vi "Controller Main Loop.vi"(8 "error in (no error)":errorcluster, 11 "msg cluster":T1) -> (0 "error out":errorcluster)   [LabVIEW 2020]
uses:
  Messaging/Messaging Cluster.ctl
  Hardware/Sensors/Cameras/Camera.lvclass
  C:/Users/Haslach/Documents/Inflation-Apparatus/src/Hardware/General Hardware.lvclass
  Hardware/Sensors/Force Sensors/Force Sensor.lvclass
  Hardware/Actuators/Servos/Servo.lvclass
  Hardware/Actuators/Switches/Switch.lvclass
  Controller Loop/Message and Data.ctl
  Inflation Test/Parameter Class/IA Test Parameters.lvclass
  Controllers/Controller.lvclass
  File Interfacing/Filename Structure.ctl
  GUI/Main GUI Loop/Handler.ctl
  Inflation Test/Result Handling/Inflation Test Numeric Results.ctl
  Controller Loop/Controller Data.ctl
  Hardware/General Hardware.lvclass/General Hardware.ctl
  Hardware/General Hardware.lvclass
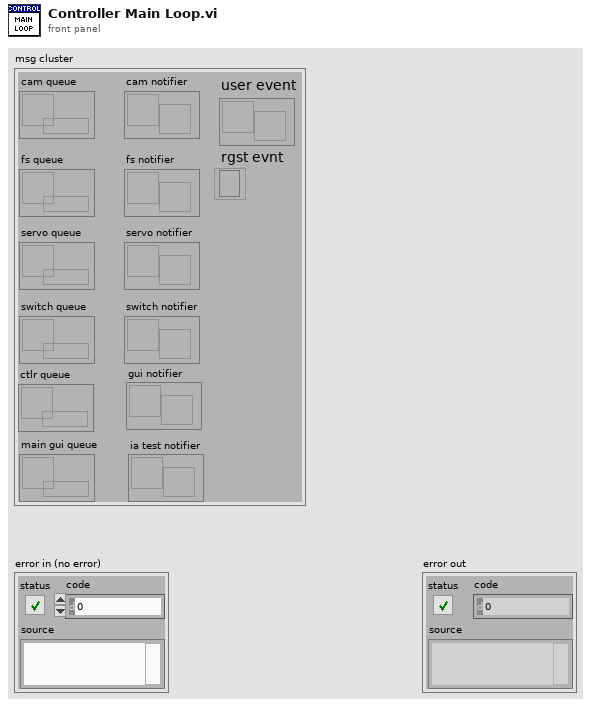
[diagram p1: front panel]
types:
  T1 = typedef "Messaging Cluster.ctl" = cluster{"cam queue":refnum<queue>, "fs queue":refnum<queue>, "servo queue":refnum<queue>, "switch queue":refnum<queue>, "switch notifier":refnum<notifier>, "servo notifier":refnum<notifier>, "fs notifier":refnum<notifier>, "cam notifier":refnum<notifier>, "rgst evnt":refnum<event-registration>, "user event":refnum<user-event>, "ctlr queue":refnum<queue>, "main gui queue":refnum<queue>, "gui notifier":refnum<notifier>, "ia test notifier":refnum<notifier>}
  T2 = typedef "Controller Data.ctl" = cluster{"diameter results":dbl[][], "force results":dbl[][], "fs cal array":dbl[][], "fs cal results":dbl[][], "start time":timestamp, "end time":timestamp, "log row":i32, "log column":i32}
  T3 = typedef "Handler.ctl" = cluster{"bool ref":refnum<vi>, "error":errorcluster, "msg":string, "status":string, "switch status":bool, "force cal":dbl[][], "force cal results":dbl[][]}
  T4 = enum32{"invalid app kind", "Development System", "Run Time System", "Student Edition", "Embedded LabVIEW", "Evaluation", "Custom"}
  T5 = typedef "Message and Data.ctl" = cluster{"msg":string, "ia test param":refnum<class "IA Test Parameters.lvclass">, "controller type":refnum<class "Controller.lvclass">, "folder path":path, "file name":string, "file comments":string, "cam":refnum<class "Camera.lvclass">, "fs":refnum<class "Force Sensor.lvclass">, "servo":refnum<class "Servo.lvclass">, "switch":refnum<class "Switch.lvclass">, "filename struct":T6}
  T6 = typedef "Filename Structure.ctl" = enum16{"<nameYYYYMMDDi>", "<name>"}
  T7 = typedef "Inflation Test Numeric Results.ctl" = cluster{"diameter":dbl, "diam time":dbl, "force":dbl, "force time":dbl, "setpoint":dbl, "servo pw":dbl, "calibration log":dbl[][], "calibration results":dbl[][]}
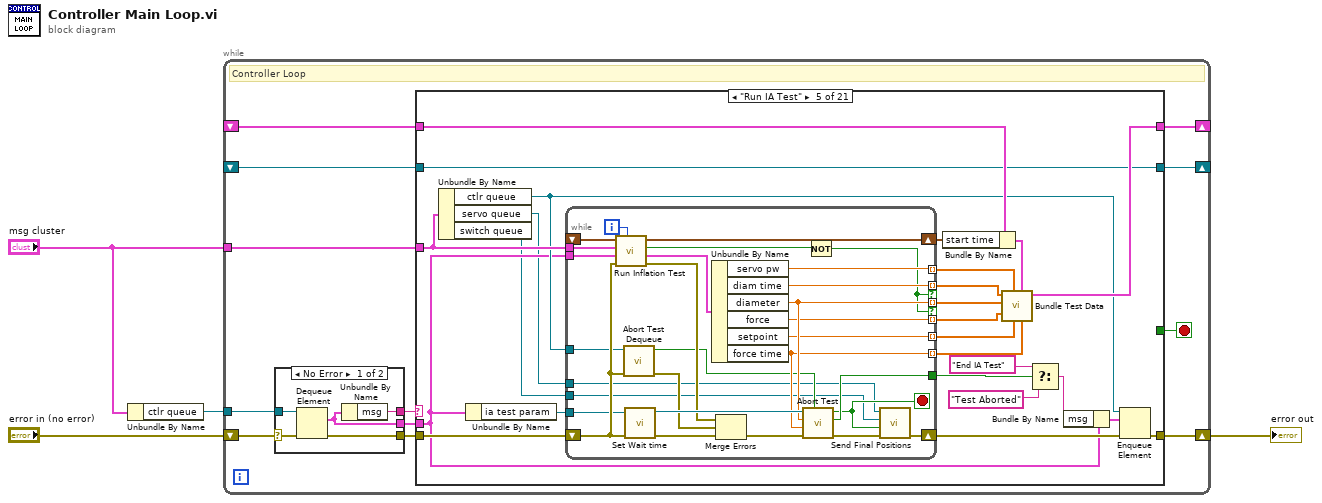
[diagram p0: block diagram]
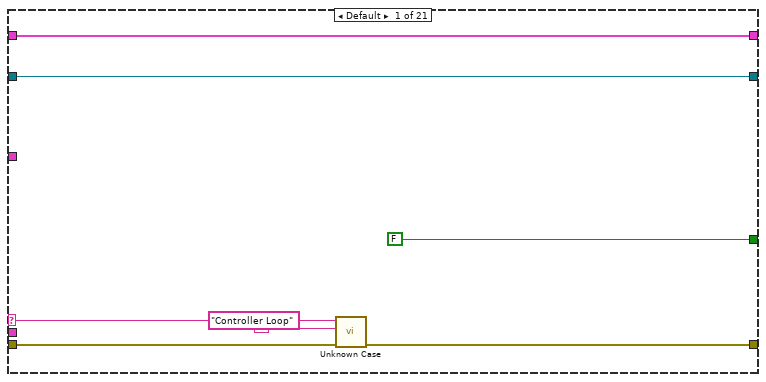
[diagram p2: hidden frame]
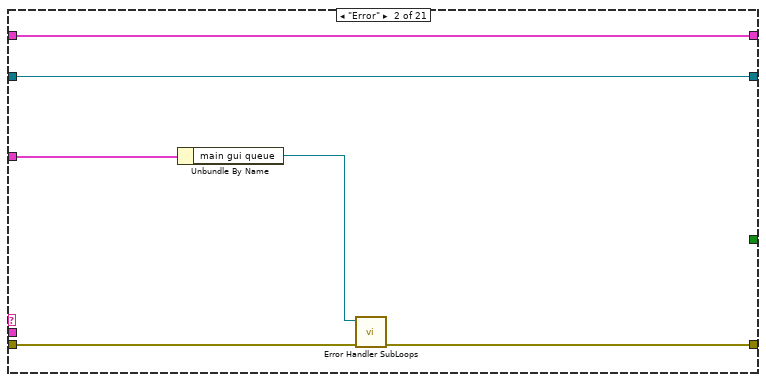
[diagram p3: hidden frame]
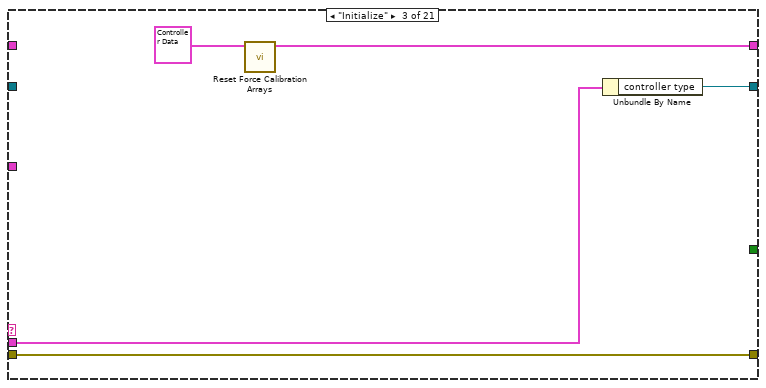
[diagram p4: hidden frame]
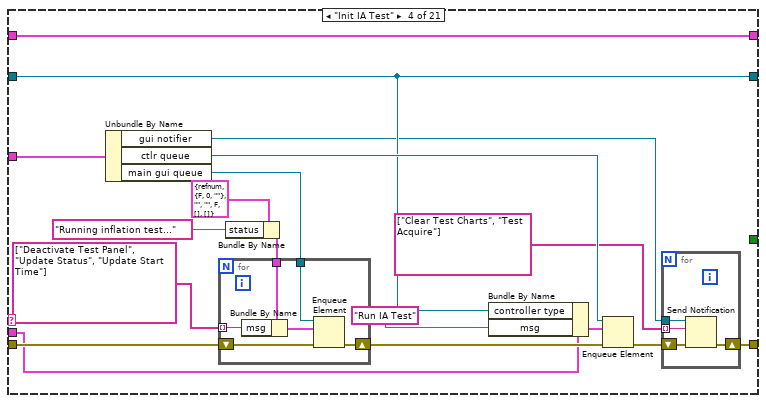
[diagram p5: hidden frame]
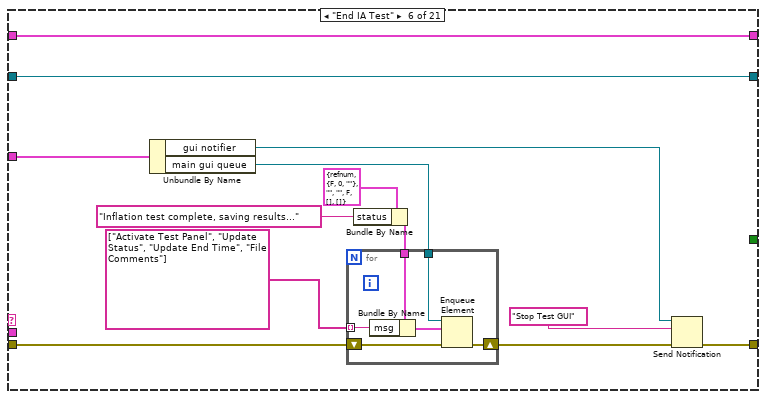
[diagram p6: hidden frame]
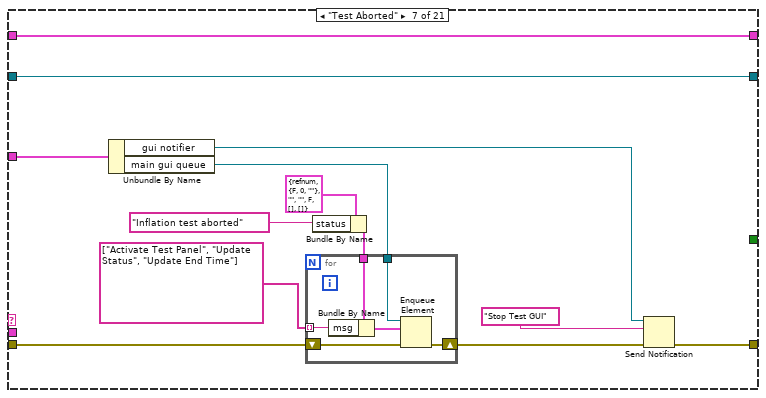
[diagram p7: hidden frame]
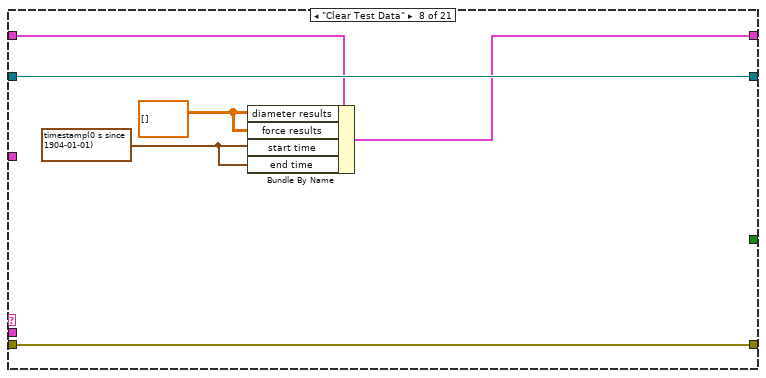
[diagram p8: hidden frame]
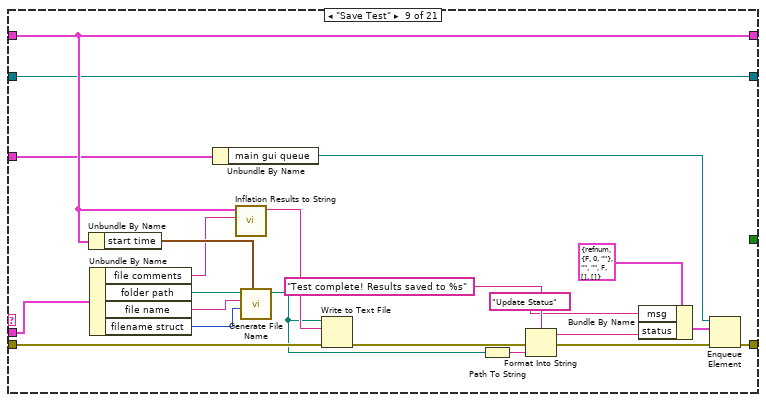
[diagram p9: hidden frame]
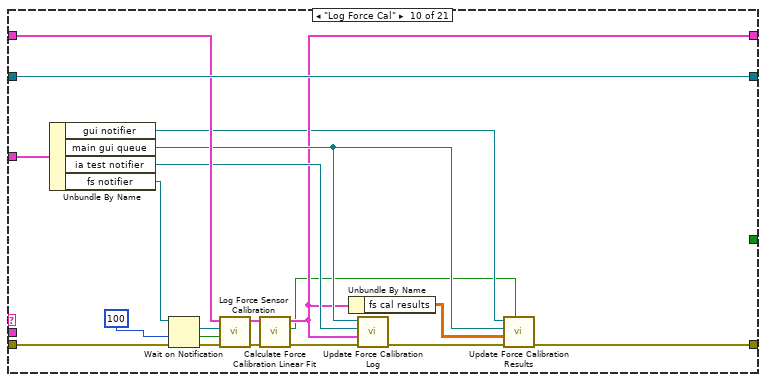
[diagram p10: hidden frame]
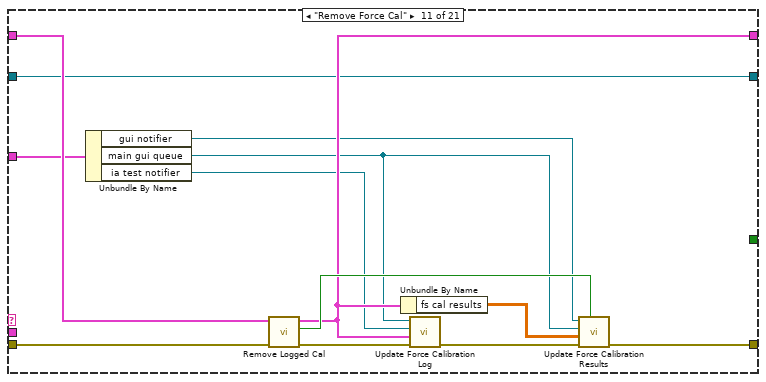
[diagram p11: hidden frame]
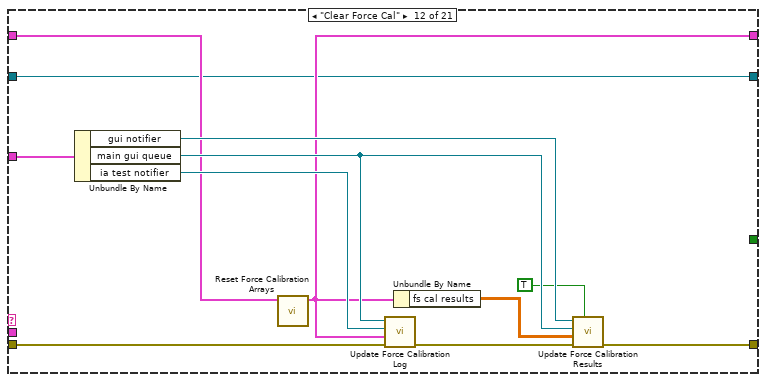
[diagram p12: hidden frame]
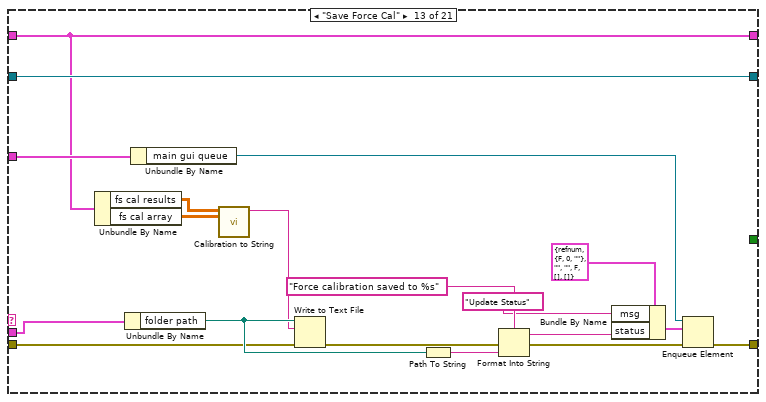
[diagram p13: hidden frame]
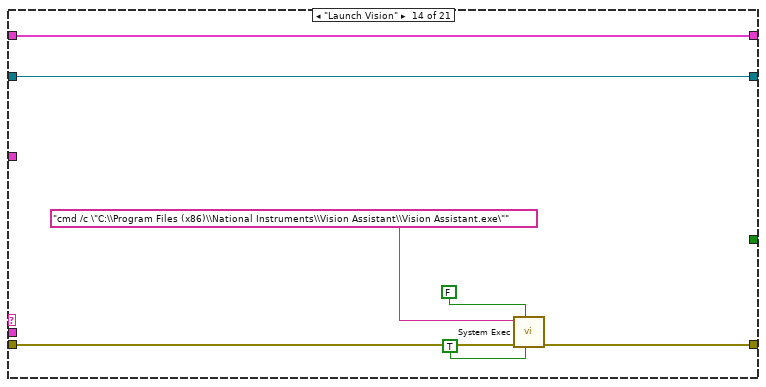
[diagram p14: hidden frame]
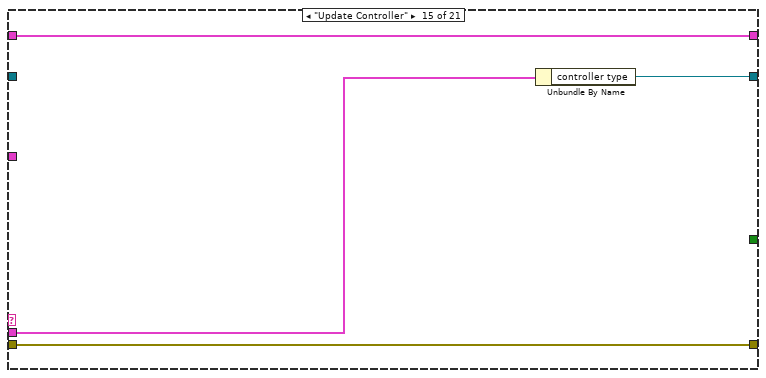
[diagram p15: hidden frame]
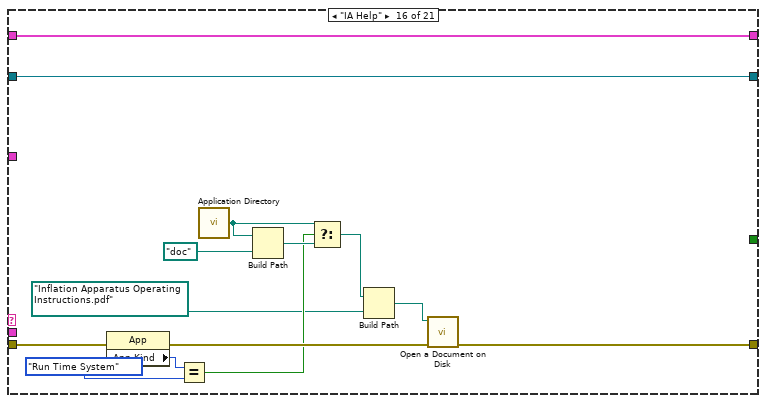
[diagram p16: hidden frame]
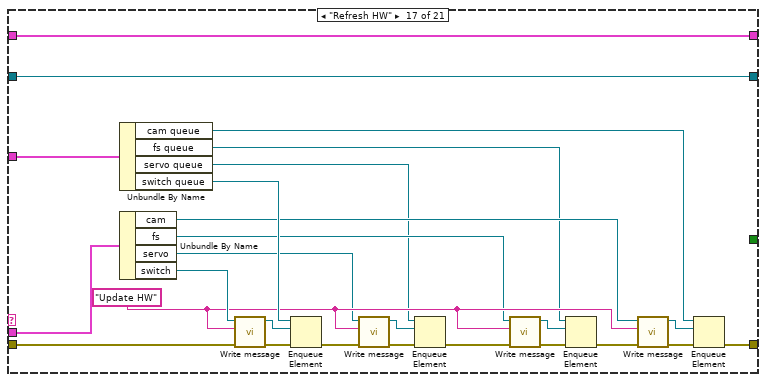
[diagram p17: hidden frame]
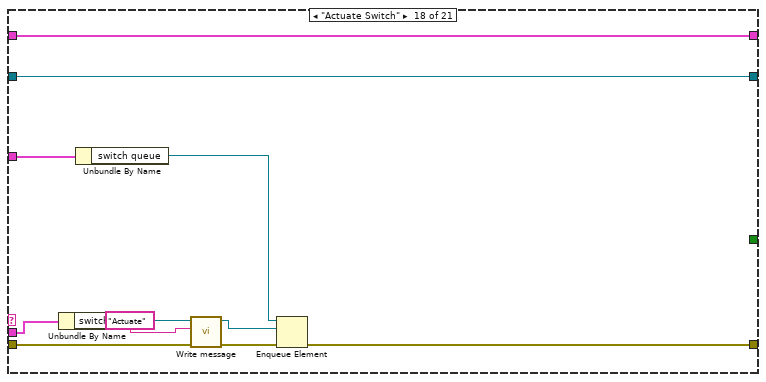
[diagram p18: hidden frame]
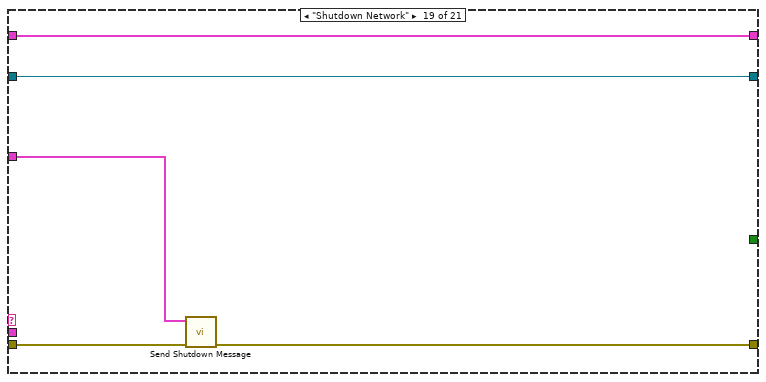
[diagram p19: hidden frame]
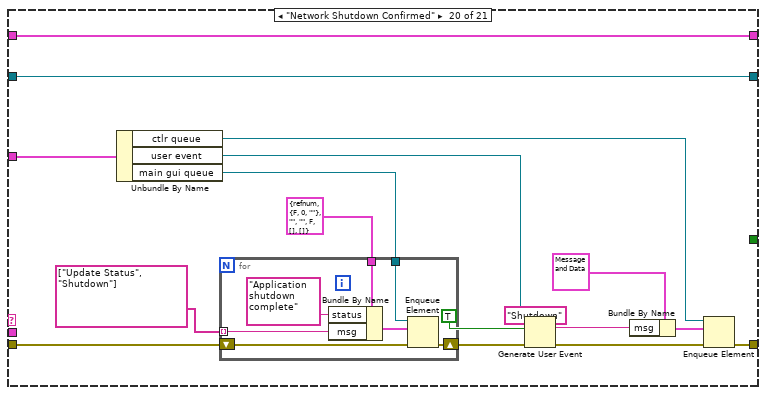
[diagram p20: hidden frame]
diagram:
  n1 = Unbundle By Name("msg cluster") -> ("ctlr queue"=w1:refnum<queue>)
  n2 = while {
    tunnel: "msg cluster" -> [w12]
    shift-right: [w14] -> w3
    shift-left: "error in (no error)" -> [w16]
    shift-right: [w8] -> _
    shift-left: _ -> [w9]
    tunnel: w1 -> [w7]
    shift-right: [w6] -> _
    shift-left: _ -> [w5]
    stop <- w11 stop-if-true
    # "Controller Loop"
    n3 = case shown="No Error" w16 {
      selector: w16 -> [w344 w348]
      tunnel: [w345 w348] -> w15
      tunnel: w7 -> [w343 _]
      tunnel: [w342 "Error" ("msg")] -> w13
      tunnel: [w341 T5 {"msg"="", "ia test param"=refnum, "controller type"=refnum, "folder path"=path "", "file name"="", "file comments"="", "cam"=refnum, "fs"=refnum, "servo"=refnum, "switch"=refnum, "filename struct"=enum."<nameYYYYMMDDi>"} ("controller loop")] -> w10
      frame No Error {
        n4 = Dequeue Element(queue=w343, error in (no error)=w344) -> (element=w341:T5, error out=w345:errorcluster)  [unwired: 1 in, 2 out]
        n5 = Unbundle By Name(w341) -> ("msg"=w342:string)
      }
      frame Error {
      }
    }
    n6 = case shown="\"Run IA Test\"" w13 {
      selector: w13 -> [w21 _ _ _ _ _ _ _ _ _ _ _ _ _ _ _ _ _ _ _ _]
      tunnel: w15 -> [w23 w26 w34 w50 w87 w125 w144 w155 w177 w199 w213 w226 w236 w250 w254 w266 w292 w303 w311 w327 w339]
      tunnel: [w22 w27 w34 w38 w72 w119 w138 w155 w167 w184 w207 w225 w230 w249 w254 w269 w279 w304 w312 w329 w339] -> w14
      tunnel: w12 -> [_ w29 _ w51 w76 w124 w143 _ w169 w202 w206 w224 w235 _ _ _ w294 w306 w313 w328 _]
      tunnel: [FALSE _ _ _ _ _ _ _ _ _ _ _ _ _ _ _ _ _ _ _ TRUE] -> w11
      tunnel: w10 -> [_ _ w33 w43 w70 _ _ _ w181 _ _ _ w238 _ w257 _ w297 w301 _ _ _]
      tunnel: w9 -> [w18 w28 _ w52 w79 w122 w141 w159 w178 w195 w211 w220 w228 w253 w255 w271 w295 w308 w310 w324 w338]
      tunnel: [w18 w28 w30 w52 w81 w122 w141 w156 w178 w187 w209 w217 w228 w253 w255 w271 w295 w308 w310 w324 w338] -> w8
      tunnel: [w17 w24 w32 w40 w75 w123 w142 w160 w175 w196 w208 w216 w229 w252 w256 w270 w296 w307 w309 w317 w337] -> w6
      tunnel: w5 -> [w17 w24 _ w40 w75 w123 w142 w160 w175 w196 w208 w216 w229 w252 _ w270 w296 w307 w309 w317 w337]
      frame Default {
        n7 = call "Unknown Case.vi"("error in (no error)"=w23, "source"="Controller Loop", "case"=w21) -> ("error out"=w22:errorcluster)  [unwired: 8 in]
      }
      frame "Error" {
        n8 = Unbundle By Name(w29) -> ("main gui queue"=w25:refnum<queue>)
        n9 = call "Error Handler SubLoops.vi"("error in"=w26, "main gui queue"=w25) -> ("error out"=w27:errorcluster)  [unwired: 9 in]
      }
      frame "Initialize" {
        n10 = call "Reset Force Calibration Arrays.vi"("array results in"=T2 {"diameter results"=[], "force results"=[], "fs cal array"=[], "fs cal results"=[], "start time"=timestamp(0 s since 1904-01-01), "end time"=timestamp(0 s since 1904-01-01), "log row"=0, "log column"=0} ("array results")) -> ("array results out"=w30:T2)  [unwired: 10 in]
        n11 = Unbundle By Name(w33) -> ("controller type"=w32:refnum<class "Controller.lvclass">)
      }
      frame "Init IA Test" {
        n12 = Unbundle By Name(w51) -> ("gui notifier"=w37:refnum<notifier>, "ctlr queue"=w44:refnum<queue>, "main gui queue"=w49:refnum<queue>)
        n13 = Bundle By Name(cluster=T3 {"bool ref"=refnum, "error"={"status"=FALSE, "code"=0, "source"=""}, "msg"="", "status"="", "switch status"=FALSE, "force cal"=[], "force cal results"=[]} ("main gui type"), "status"="Running inflation test...") -> (w46:T3)
        n14 = for {
          tunnel: w46 -> [w61]
          tunnel: w49 -> [w58]
          shift-right: [w60] -> w45
          shift-left: w50 -> [w62]
          tunnel: string[] ["Deactivate Test Panel", "Update Status", "Update Start Time"] ("msg") -> [w57] mode=indexing
          n15 = Bundle By Name(cluster=w61, "msg"=w57) -> (w59:T3)
          n16 = Enqueue Element(queue=w58, element=w59, error in (no error)=w62) -> (error out=w60:errorcluster)  [unwired: 1 in, 2 out]
        }
        n17 = Bundle By Name(cluster=w43, "controller type"=w40, "msg"="Run IA Test") -> (w42:T5)
        n18 = Enqueue Element(queue=w44, element=w42, error in (no error)=w45) -> (error out=w39:errorcluster)  [unwired: 1 in, 2 out]
        n19 = for {
          tunnel: w37 -> [w54]
          tunnel: string[] ["Clear Test Charts", "Test Acquire"] ("notification") -> [w53] mode=indexing
          shift-right: [w55] -> w38
          shift-left: w39 -> [w56]
          n20 = Send Notification(notification=w53, notifier=w54, error in (no error)=w56) -> (error out=w55:errorcluster)  [unwired: 1 out]
        }
      }
      frame "Run IA Test" {
        n21 = Unbundle By Name(w76) -> ("ctlr queue"=w71:refnum<queue>, "servo queue"=w63:refnum<queue>, "switch queue"=w64:refnum<queue>)
        n22 = Unbundle By Name(w70) -> ("ia test param"=w74:refnum<class "IA Test Parameters.lvclass">)
        n23 = while {
          tunnel: w76 -> [w109]
          tunnel: w70 -> [w112]
          shift-right: [w111] -> w78
          shift-left: _ -> [w110]
          shift-right: [w91] -> w73
          shift-left: w87 -> [w101]
          tunnel: [w107] -> w82 mode=indexing if=w93
          tunnel: [w106] -> w83 mode=indexing if=w93
          tunnel: [w105] -> w84 mode=indexing
          tunnel: [w104] -> w85 mode=indexing
          tunnel: [w103] -> w86 mode=indexing
          tunnel: [w102] -> w80 mode=indexing
          tunnel: w71 -> [w97]
          tunnel: w74 -> [w96]
          tunnel: [w95] -> w65
          tunnel: w64 -> [w88]
          tunnel: w63 -> [w89]
          i -> [w116]
          stop <- w90 stop-if-true
          n24 = call "Run Inflation Test.vi"("iteration"=w116, "error in (no error)"=w101, "controller data"=w112, "msg network"=w109, "start time in"=w110) -> ("error out"=w100:errorcluster, "ia test data"=w108:T7, "cam timed out?"=w94:bool, "start time out"=w111:timestamp)  [unwired: 2 in, 1 out]
          n25 = call "Abort Test Dequeue.vi"("error in (no error)"=w101, "ctlr queue"=w97) -> ("error out"=w99:errorcluster, "abort?"=w98:bool)  [unwired: 8 in]
          n26 = call "Set Wait time.vi"("error in (no error)"=w101, "ia test param in"=w96) -> ("error out"=w114:errorcluster, "ia test param out"=w115:refnum<class "IA Test Parameters.lvclass">)  [unwired: 8 in]
          n27 = Unbundle By Name(w108) -> ("servo pw"=w102:dbl, "diam time"=w107:dbl, "diameter"=w106:dbl, "force"=w105:dbl, "setpoint"=w104:dbl, "force time"=w103:dbl)
          n28 = Merge Errors(w100, w99, w114) -> (w113:errorcluster)
          n29 = call "Abort Test.vi"("abort test?"=w98, "error in (no error)"=w113, "time (sec)"=w103, "diameter (mm)"=w106, "IA Test Parameters in"=w115) -> ("error out"=w92:errorcluster, "test completed?"=w95:bool, "end test?"=w90:bool)  [unwired: 4 in]
          n30 = Not(x=w94) -> (.not. x?=w93:bool)
          n31 = call "Send Final Positions.vi"("error in (no error)"=w92, "end test?"=w90, "switch queue"=w88, "Queue in"=w89) -> ("error out"=w91:errorcluster)  [unwired: 7 in]
        }
        n32 = Bundle By Name(cluster=w79, "start time"=w78) -> (w77:T2)
        n33 = call "Bundle Test Data.vi"("force time"=w86, "array results in"=w77, "setpoint"=w85, "servo pw"=w80, "force"=w84, "diameter"=w83, "diameter time"=w82) -> ("array results out"=w81:T2)  [unwired: 4 in]
        n34 = Select(t="End IA Test" ("msg"), s=w65, f="Test Aborted" ("msg")) -> (s? t:f=w67:string)
        n35 = Bundle By Name(cluster=w70, "msg"=w67) -> (w69:T5)
        n36 = Enqueue Element(queue=w71, element=w69, error in (no error)=w73) -> (error out=w72:errorcluster)  [unwired: 1 in, 2 out]
      }
      frame "End IA Test" {
        n37 = Unbundle By Name(w124) -> ("gui notifier"=w118:refnum<notifier>, "main gui queue"=w129:refnum<queue>)
        n38 = Bundle By Name(cluster=T3 {"bool ref"=refnum, "error"={"status"=FALSE, "code"=0, "source"=""}, "msg"="", "status"="", "switch status"=FALSE, "force cal"=[], "force cal results"=[]} ("main gui type"), "status"="Inflation test complete, saving results...") -> (w126:T3)
        n39 = for {
          tunnel: w126 -> [w134]
          tunnel: w129 -> [w131]
          shift-right: [w133] -> w120
          shift-left: w125 -> [w135]
          tunnel: string[] ["Activate Test Panel", "Update Status", "Update End Time", "File Comments"] ("msg") -> [w130] mode=indexing
          n40 = Bundle By Name(cluster=w134, "msg"=w130) -> (w132:T3)
          n41 = Enqueue Element(queue=w131, element=w132, error in (no error)=w135) -> (error out=w133:errorcluster)  [unwired: 1 in, 2 out]
        }
        n42 = Send Notification(notification="Stop Test GUI", notifier=w118, error in (no error)=w120) -> (error out=w119:errorcluster)  [unwired: 1 out]
      }
      frame "Test Aborted" {
        n43 = Unbundle By Name(w143) -> ("gui notifier"=w137:refnum<notifier>, "main gui queue"=w147:refnum<queue>)
        n44 = Bundle By Name(cluster=T3 {"bool ref"=refnum, "error"={"status"=FALSE, "code"=0, "source"=""}, "msg"="", "status"="", "switch status"=FALSE, "force cal"=[], "force cal results"=[]} ("main gui type"), "status"="Inflation test aborted") -> (w148:T3)
        n45 = for {
          tunnel: w148 -> [w153]
          tunnel: w147 -> [w150]
          shift-right: [w152] -> w139
          shift-left: w144 -> [w154]
          tunnel: string[] ["Activate Test Panel", "Update Status", "Update End Time"] ("msg") -> [w149] mode=indexing
          n46 = Bundle By Name(cluster=w153, "msg"=w149) -> (w151:T3)
          n47 = Enqueue Element(queue=w150, element=w151, error in (no error)=w154) -> (error out=w152:errorcluster)  [unwired: 1 in, 2 out]
        }
        n48 = Send Notification(notification="Stop Test GUI", notifier=w137, error in (no error)=w139) -> (error out=w138:errorcluster)  [unwired: 1 out]
      }
      frame "Clear Test Data" {
        w157 = timestamp(0 s since 1904-01-01) ("start time")
        w158 = dbl[][] [] ("diameter results")
        n49 = Bundle By Name(cluster=w159, "diameter results"=w158, "force results"=w158, "start time"=w157, "end time"=w157) -> (w156:T2)
      }
      frame "Save Test" {
        n50 = Unbundle By Name(w178) -> ("start time"=w182:timestamp)
        n51 = Unbundle By Name(w181) -> ("file comments"=w174:string, "folder path"=w180:path, "file name"=w179:string, "filename struct"=w161:T6)
        n52 = Unbundle By Name(w169) -> ("main gui queue"=w166:refnum<queue>)
        n53 = call "Inflation Results to String.vi"("comments"=w174, "results"=w178) -> ("Results String"=w176:string)  [unwired: 9 in]
        n54 = call "Generate File Name.vi"("Time Stamp"=w182, "filename struct"=w161, "Test Name"=w179, "Folder Location"=w180) -> ("Generated File Path"=w170:path)  [unwired: 7 in]
        n55 = Write to Text File(file (use dialog)=w170, text=w176, error in=w177) -> (error out=w171:errorcluster)  [unwired: 1 in, 2 out]
        n56 = Path To String(path=w170) -> (string=w172:string)
        n57 = Format Into String(format string="Test complete! Results saved to %s", error in=w171, w172) -> (resulting string=w163:string, error out=w168:errorcluster)  [unwired: 1 in]
        n58 = Bundle By Name(cluster=T3 {"bool ref"=refnum, "error"={"status"=FALSE, "code"=0, "source"=""}, "msg"="", "status"="", "switch status"=FALSE, "force cal"=[], "force cal results"=[]} ("element"), "msg"="Update Status", "status"=w163) -> (w164:T3)
        n59 = Enqueue Element(queue=w166, element=w164, error in (no error)=w168) -> (error out=w167:errorcluster)  [unwired: 1 in, 2 out]
      }
      frame "Log Force Cal" {
        n60 = Unbundle By Name(w202) -> ("gui notifier"=w185:refnum<notifier>, "main gui queue"=w188:refnum<queue>, "ia test notifier"=w190:refnum<notifier>, "fs notifier"=w201:refnum<notifier>)
        n61 = Wait on Notification(notifier=w201, timeout in ms (-1)=100, error in (no error)=w199) -> (notification=w194:refnum<class "Force Sensor.lvclass">, timed out?=w197:bool, error out=w198:errorcluster)  [unwired: 1 in, 1 out]
        n62 = call "Log Force Sensor Calibration.vi"("error in (no error)"=w198, "timed out?"=w197, "Force Sensor in"=w194, "array results in"=w195) -> ("error out"=w192:errorcluster, "array results out"=w193:T2)  [unwired: 6 in]
        n63 = call "Calculate Force Calibration Linear Fit.vi"("error in (no error)"=w192, "array results in"=w193) -> ("error out"=w191:errorcluster, "new results?"=w183:bool, "array results out"=w187:T2)  [unwired: 7 in]
        n64 = Unbundle By Name(w187) -> ("fs cal results"=w186:dbl[][])
        n65 = call "Update Force Calibration Log.vi"("error in (no error)"=w191, "array results in"=w187, "ia test notifier"=w190, "main gui queue"=w188) -> ("error out"=w189:errorcluster)  [unwired: 7 in]
        n66 = call "Update Force Calibration Results.vi"("new results?"=w183, "error in (no error)"=w189, "fs cal results"=w186, "main gui queue"=w188, "gui notifier"=w185) -> ("error out"=w184:errorcluster)  [unwired: 6 in]
      }
      frame "Remove Force Cal" {
        n67 = Unbundle By Name(w206) -> ("gui notifier"=w203:refnum<notifier>, "main gui queue"=w204:refnum<queue>, "ia test notifier"=w205:refnum<notifier>)
        n68 = call "Remove Logged Cal.vi"("error in (no error)"=w213, "array results in"=w211) -> ("error out"=w212:errorcluster, "update results?"=w210:bool, "array results out"=w209:T2)  [unwired: 7 in]
        n69 = Unbundle By Name(w209) -> ("fs cal results"=w214:dbl[][])
        n70 = call "Update Force Calibration Log.vi"("error in (no error)"=w212, "array results in"=w209, "ia test notifier"=w205, "main gui queue"=w204) -> ("error out"=w215:errorcluster)  [unwired: 7 in]
        n71 = call "Update Force Calibration Results.vi"("new results?"=w210, "error in (no error)"=w215, "fs cal results"=w214, "main gui queue"=w204, "gui notifier"=w203) -> ("error out"=w207:errorcluster)  [unwired: 6 in]
      }
      frame "Clear Force Cal" {
        n72 = Unbundle By Name(w224) -> ("gui notifier"=w222:refnum<notifier>, "main gui queue"=w221:refnum<queue>, "ia test notifier"=w223:refnum<notifier>)
        n73 = call "Reset Force Calibration Arrays.vi"("array results in"=w220) -> ("array results out"=w217:T2)  [unwired: 10 in]
        n74 = call "Update Force Calibration Log.vi"("error in (no error)"=w226, "array results in"=w217, "ia test notifier"=w223, "main gui queue"=w221) -> ("error out"=w227:errorcluster)  [unwired: 7 in]
        n75 = Unbundle By Name(w217) -> ("fs cal results"=w219:dbl[][])
        n76 = call "Update Force Calibration Results.vi"("new results?"=TRUE, "error in (no error)"=w227, "fs cal results"=w219, "main gui queue"=w221, "gui notifier"=w222) -> ("error out"=w225:errorcluster)  [unwired: 6 in]
      }
      frame "Save Force Cal" {
        n77 = Unbundle By Name(w228) -> ("fs cal results"=w232:dbl[][], "fs cal array"=w233:dbl[][])
        n78 = Unbundle By Name(w238) -> ("folder path"=w237:path)
        n79 = Unbundle By Name(w235) -> ("main gui queue"=w234:refnum<queue>)
        n80 = call "Calibration to String.vi"("fs cal array"=w233, "fs cal results"=w232) -> ("cal string"=w231:string)  [unwired: 9 in]
        n81 = Write to Text File(file (use dialog)=w237, text=w231, error in=w236) -> (error out=w244:errorcluster)  [unwired: 1 in, 2 out]
        n82 = Path To String(path=w237) -> (string=w245:string)
        n83 = Format Into String(format string="Force calibration saved to %s", error in=w244, w245) -> (resulting string=w240:string, error out=w243:errorcluster)  [unwired: 1 in]
        n84 = Bundle By Name(cluster=T3 {"bool ref"=refnum, "error"={"status"=FALSE, "code"=0, "source"=""}, "msg"="", "status"="", "switch status"=FALSE, "force cal"=[], "force cal results"=[]} ("element"), "msg"="Update Status", "status"=w240) -> (w241:T3)
        n85 = Enqueue Element(queue=w234, element=w241, error in (no error)=w243) -> (error out=w230:errorcluster)  [unwired: 1 in, 2 out]
      }
      frame "Launch Vision" {
        n86 = call <vilib>:"System Exec.vi"("run minimized? (F)"=TRUE, "wait until completion? (T)"=FALSE, "error in (no error)"=w250, "command line"="cmd /c \"C:\\Program Files (x86)\\National Instruments\\Vision Assistant\\Vision Assistant.exe\"") -> ("error out"=w249:errorcluster)  [unwired: 4 in, 3 out]
      }
      frame "Update Controller" {
        n87 = Unbundle By Name(w257) -> ("controller type"=w256:refnum<class "Controller.lvclass">)
      }
      frame "IA Help" {
        n88 = property class="App"(error in=w266) -> (error out=w265:errorcluster, "App.Kind"=w267:T4)  [unwired: 1 in, 1 out]
        n89 = Equal?(x=w267, y=T4."Run Time System" ("Application:Kind")) -> (x = y?=w261:bool)
        n90 = call <vilib>:"Application Directory.vi"() -> ("Application Directory"=w262:path)
        n91 = Build Path(base path=w262, name or relative path=path "doc" ("Path")) -> (appended path=w263:path)
        n92 = Select(t=w262, s=w261, f=w263) -> (s? t:f=w260:path)
        n93 = Build Path(base path=w260, name or relative path=path "Inflation Apparatus Operating Instructions.pdf" ("Path")) -> (appended path=w258:path)
        n94 = call "Open a Document on Disk.vi"("error in (no error)"=w265, "document path"=w258) -> ("error out"=w269:errorcluster)  [unwired: 5 in]
      }
      frame "Refresh HW" {
        w278 = "Update HW"
        n95 = Unbundle By Name(w294) -> ("cam queue"=w272:refnum<queue>, "fs queue"=w273:refnum<queue>, "servo queue"=w274:refnum<queue>, "switch queue"=w293:refnum<queue>)
        n96 = Unbundle By Name(w297) -> ("cam"=w275:refnum<class "Camera.lvclass">, "fs"=w276:refnum<class "Force Sensor.lvclass">, "servo"=w277:refnum<class "Servo.lvclass">, "switch"=w290:refnum<class "Switch.lvclass">)
        n97 = call "Write message.vi"("error in (no error)"=w292, "message"=w278, "General Hardware in"=w290) -> ("error out"=w291:errorcluster, "General Hardware out"=w289:refnum<class "Switch.lvclass">)  [unwired: 7 in]
        n98 = Enqueue Element(queue=w293, element=w289, error in (no error)=w291) -> (error out=w282:errorcluster)  [unwired: 1 in, 2 out]
        n99 = call "Write message.vi"("error in (no error)"=w282, "message"=w278, "General Hardware in"=w277) -> ("error out"=w288:errorcluster, "General Hardware out"=w287:refnum<class "Servo.lvclass">)  [unwired: 7 in]
        n100 = Enqueue Element(queue=w274, element=w287, error in (no error)=w288) -> (error out=w281:errorcluster)  [unwired: 1 in, 2 out]
        n101 = call "Write message.vi"("error in (no error)"=w281, "message"=w278, "General Hardware in"=w276) -> ("error out"=w286:errorcluster, "General Hardware out"=w285:refnum<class "Force Sensor.lvclass">)  [unwired: 7 in]
        n102 = Enqueue Element(queue=w273, element=w285, error in (no error)=w286) -> (error out=w280:errorcluster)  [unwired: 1 in, 2 out]
        n103 = call "Write message.vi"("error in (no error)"=w280, "message"=w278, "General Hardware in"=w275) -> ("error out"=w284:errorcluster, "General Hardware out"=w283:refnum<class "Camera.lvclass">)  [unwired: 7 in]
        n104 = Enqueue Element(queue=w272, element=w283, error in (no error)=w284) -> (error out=w279:errorcluster)  [unwired: 1 in, 2 out]
      }
      frame "Actuate Switch" {
        n105 = Unbundle By Name(w301) -> ("switch"=w300:refnum<class "Switch.lvclass">)
        n106 = Unbundle By Name(w306) -> ("switch queue"=w305:refnum<queue>)
        n107 = call "Write message.vi"("error in (no error)"=w303, "message"="Actuate", "General Hardware in"=w300) -> ("error out"=w302:errorcluster, "General Hardware out"=w298:refnum<class "Switch.lvclass">)  [unwired: 7 in]
        n108 = Enqueue Element(queue=w305, element=w298, error in (no error)=w302) -> (error out=w304:errorcluster)  [unwired: 1 in, 2 out]
      }
      frame "Shutdown Network" {
        n109 = call "Send Shutdown Message.vi"("error in (no error)"=w311, "msg cluster"=w313) -> ("error out"=w312:errorcluster)  [unwired: 9 in]
      }
      frame "Network Shutdown Confirmed" {
        n110 = Unbundle By Name(w328) -> ("ctlr queue"=w322:refnum<queue>, "user event"=w319:refnum<user-event>, "main gui queue"=w326:refnum<queue>)
        n111 = for {
          tunnel: w326 -> [w334]
          tunnel: T3 {"bool ref"=refnum, "error"={"status"=FALSE, "code"=0, "source"=""}, "msg"="", "status"="", "switch status"=FALSE, "force cal"=[], "force cal results"=[]} ("main gui type") -> [w333]
          shift-right: [w335] -> w321
          shift-left: w327 -> [w336]
          tunnel: string[] ["Update Status", "Shutdown"] -> [w330] mode=indexing
          n112 = Bundle By Name(cluster=w333, "status"="Application shutdown complete", "msg"=w330) -> (w332:T3)
          n113 = Enqueue Element(queue=w334, element=w332, error in (no error)=w336) -> (error out=w335:errorcluster)  [unwired: 1 in, 2 out]
        }
        n114 = Generate User Event(user event=w319, event data cluster=TRUE ("event data"), error in=w321) -> (error out=w320:errorcluster)  [unwired: 1 in, 1 out]
        n115 = Bundle By Name(cluster=T5 {"msg"="", "ia test param"=refnum, "controller type"=refnum, "folder path"=path "", "file name"="", "file comments"="", "cam"=refnum, "fs"=refnum, "servo"=refnum, "switch"=refnum, "filename struct"=enum."<nameYYYYMMDDi>"} ("element"), "msg"="Shutdown") -> (w315:T5)
        n116 = Enqueue Element(queue=w322, element=w315, error in (no error)=w320) -> (error out=w329:errorcluster)  [unwired: 1 in, 2 out]
      }
      frame "Shutdown" {
      }
    }
  }
  "error out" <- w3
